vi "000Main V180214.vi"() -> ()   [LabVIEW 2015]
uses:
  0254/BrooksDLL64.dll
panel:
  out "Function Output Comment 4":string
  out "output param 4":i32
  out "Function Output Comment 3":string
  out "output param 3":i32
  in  "0254 Decimal Place 3":i32(ring) items=["xxx.", "xx.x", "x.xx", ".xxx"]
  out "Function Output Comment 5":string
  out "output param 5":i32
  in  "0254 Decimal Place 4":i32(ring) items=["xxx.", "xx.x", "x.xx", ".xxx"]
  out "Function Output Comment 6":string
  out "output param 6":i32
  out "resistance":cluster{dbl[], dbl[]}(graph)
  out "current":cluster{dbl[], dbl[]}(graph)
  out "flow2":cluster{dbl[], dbl[]}(graph)
  in  "?":enum32{"initialization", "step", "other"}(tab)
  in  "Start_2400":bool
  in  "Delay (ms)":u32=1000
  in  "Target (V)":dbl=0.1
  in  "Step (V)":dbl=0.005
  in  "Stop":bool
  in  "file path (use dialog)":path
  in  "?":bool
  in  "sum flow 2":dbl=100.0 format="%#_13g"
  in  "VISA 0254":refnum<visa-resource-name>
  in  "VISA 2400":refnum<visa-resource-name>
  in  "Gas Flow Enable":bool
  in  "flow2 1":dbl=100.0 format="%#_13g"
  in  "time1":dbl=1000.0 format="%#_13g"
  in  "flow2 2":dbl format="%#_13g"
  in  "time2":dbl=1000.0 format="%#_13g"
  in  "flow2 3":dbl=100.0 format="%#_13g"
  in  "time3":dbl=1000.0 format="%#_13g"
  in  "time4":dbl=1000.0 format="%#_13g"
  out "voltage":string
  out "Current":dbl
  out "Time (s)":dbl
  out "flow1":sgl format="%.2f"
  out "flow2":sgl format="%.2f"
  out "Initiliazation Started":bool
  in  "Initialization":bool
  # "flow2 = 0"
  # "flow2 = 0"
  # "time   voltage  current  flow1  flow2  resistance"
  # "Please Wait  ~ 25 s"
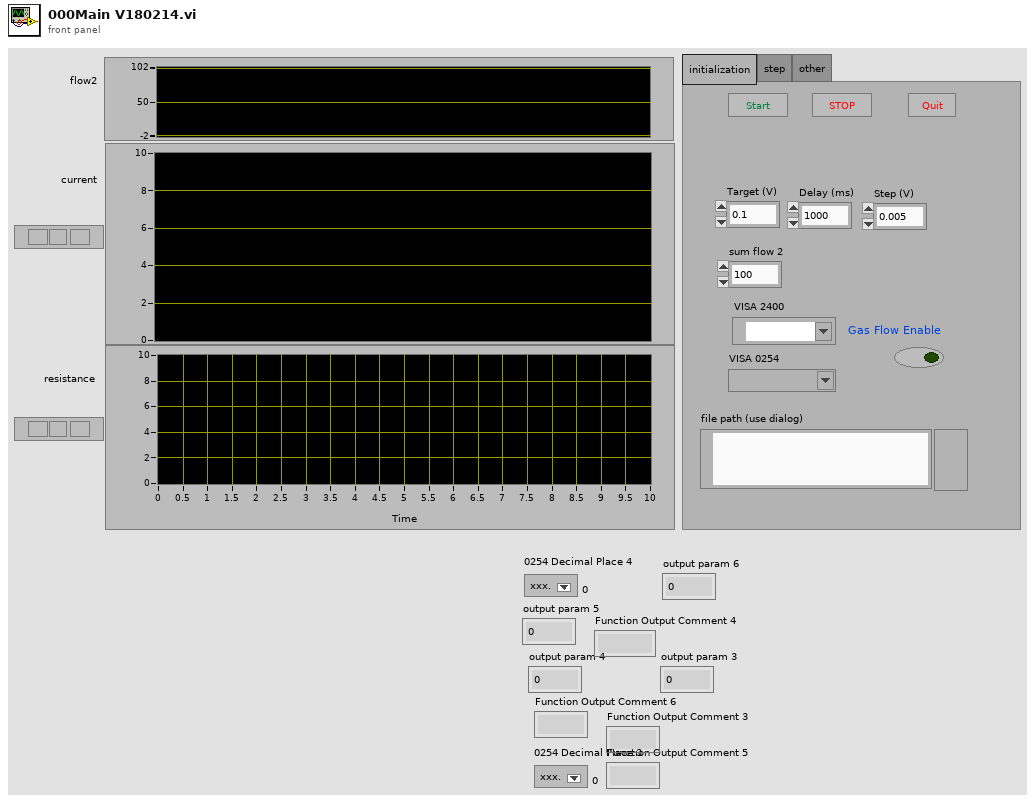
[diagram p1: front panel]
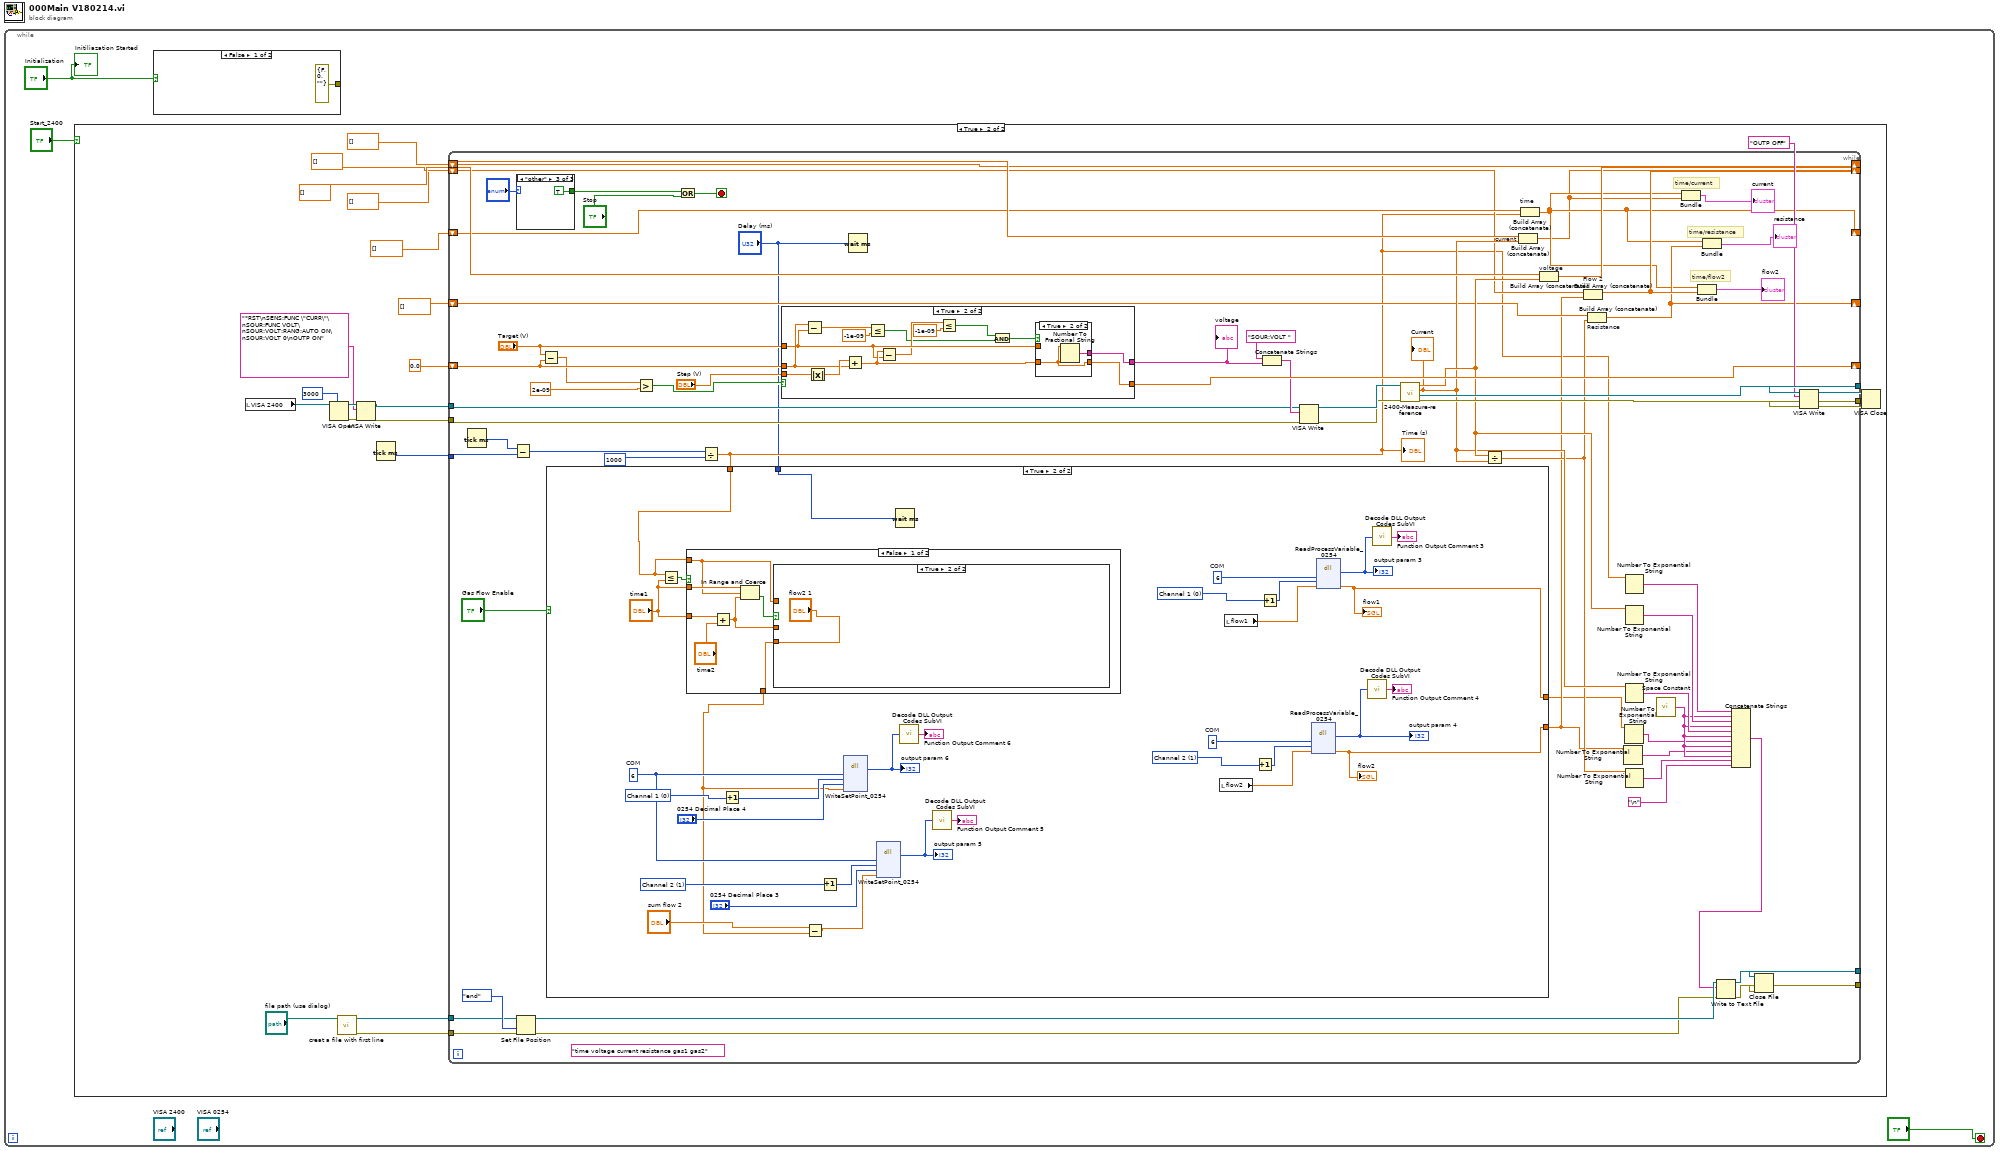
[diagram p0: block diagram]
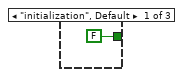
[diagram p3: hidden frame]
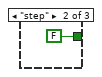
[diagram p4: hidden frame]
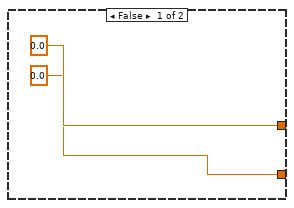
[diagram p5: hidden frame]
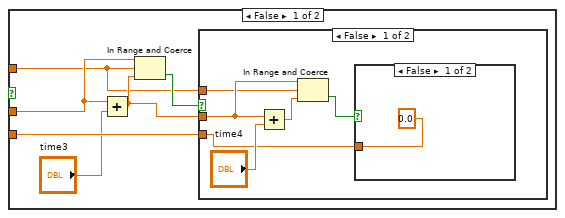
[diagram p6: hidden frame]
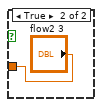
[diagram p7: hidden frame]
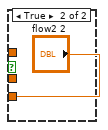
[diagram p8: hidden frame]
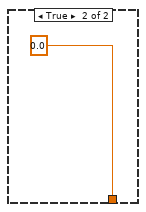
[diagram p9: hidden frame]
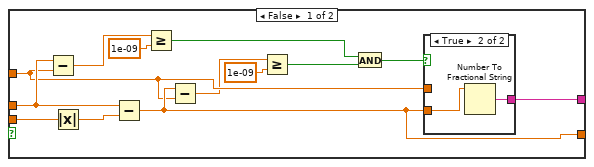
[diagram p10: hidden frame]
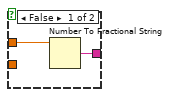
[diagram p11: hidden frame]
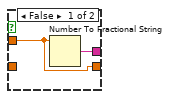
[diagram p12: hidden frame]
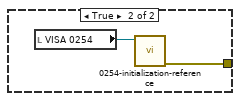
[diagram p13: hidden frame]
diagram:
  n1 = while {
    stop <- "?" stop-if-true
    n2 = case shown="True" "Start_2400" {
      frame False {
      }
      frame True {
        n3 = local read "VISA 2400"() -> (w20:refnum<visa-resource-name>)
        n4 = VISA Open(timeout (0)=3000 ("timeout ms (488.2 global)"), VISA resource name=w20) -> (VISA resource name=w23:refnum<visa-resource-name>, error out=w22:errorcluster)  [unwired: 3 in]
        n5 = call "creat a file with first line.vi"("file path (use dialog)"="file path (use dialog)") -> ("error out"=w5:errorcluster, "Byte Stream File out"=w6:refnum<file>)  [unwired: 9 in]
        n6 = VISA Write(VISA resource name=w23, write buffer="*RST\nSENS:FUNC \"CURR\"\nSOUR:FUNC VOLT\nSOUR:VOLT:RANG:AUTO ON\nSOUR:VOLT 0\nOUTP ON" ("data"), error in (no error)=w22) -> (VISA resource name out=w17:refnum<visa-resource-name>, error out=w18:errorcluster)  [unwired: 1 out]
        n7 = Tick Count (ms)() -> (millisecond timer value=w4:u32)
        n8 = while {
          shift-right: [w80] -> _
          shift-left: 0.0 ("Target (V)") -> [w76]
          shift-right: [w47] -> _
          shift-left: dbl[] [] -> [w89]
          shift-right: [w42] -> _
          shift-left: dbl[] [] -> [w88]
          tunnel: w6 -> [w41]
          tunnel: w5 -> [w85]
          tunnel: [w65] -> w26
          tunnel: [w50] -> w25
          tunnel: w17 -> [w72]
          tunnel: [w61] -> w13
          tunnel: [w60] -> w12
          tunnel: w18 -> [w66]
          tunnel: w4 -> [w37]
          shift-right: [w43] -> _
          shift-left: dbl[] [] -> [w67]
          shift-right: [w48] -> _
          shift-left: dbl[] [] -> [w49]
          shift-right: [w46] -> _
          shift-left: dbl[] [] -> [w46]
          shift-right: [w44] -> _
          shift-left: dbl[] [] -> [w45]
          stop <- w55 stop-if-true
          (unwired) "time voltage current resistance gas1 gas2"
          # "time/flow2"
          # "time/resistance"
          # "time/current"
          n9 = Tick Count (ms)() -> (millisecond timer value=w70:u32)
          n10 = Subtract(x=w70, y=w37) -> (x-y=w69:u32)
          n11 = case shown="\"other\"" "?" {
            tunnel: [FALSE FALSE TRUE] -> w57
            frame "initialization", Default {
            }
            frame "step" {
            }
            frame "other" {
            }
          }
          n12 = Set File Position(refnum=w41, from (0:start)=enum16{"start", "end", "current"}."end", error in=w85) -> (refnum out=w84:refnum<file>, error out=w83:errorcluster)  [unwired: 1 out]
          n13 = Subtract(x="Target (V)", y=w76) -> (x-y=w75:dbl)
          n14 = Greater?(x=w75, y=2e-09) -> (0:w79:bool)
          n15 = Or(x=w57, y="Stop") -> (x .or. y?=w55:bool)
          n16 = Divide(x=w69, y=u32 1000) -> (x/y=w33:dbl)
          "Time (s)" <- w33
          n17 = case shown="True" "Gas Flow Enable" {
            tunnel: [sgl 0.0 ("PV") w126] -> w35
            tunnel: [sgl 0.0 ("PV") w127] -> w34
            tunnel: w33 -> [_ w125]
            tunnel: "Delay (ms)" -> [_ w96]
            frame False {
            }
            frame True {
              w99 = 1 items=["Channel 1", "Channel 2", "Channel 3", "Channel 4"] ("0254 Channel (1-4)")
              w103 = 6  # COM
              w105 = 0 items=["Channel 1", "Channel 2", "Channel 3", "Channel 4"] ("0254 Channel (1-4)")
              w109 = 6  # COM
              w122 = 0 items=["Channel 1", "Channel 2", "Channel 3", "Channel 4"] ("0254 Channel (1-4)")
              w118 = 1 items=["Channel 1", "Channel 2", "Channel 3", "Channel 4"] ("0254 Channel 2")
              w113 = 6  # COM
              n18 = Less Or Equal?(x=w125, y="time1") -> (x <= y?=w110:bool)
              n19 = case shown="False" w110 {
                tunnel: [w132 0.0 ("flow2 2")] -> w111
                tunnel: w125 -> [w130 _]
                tunnel: "time1" -> [w134 _]
                tunnel: "time1" -> [w128 _]
                frame False {
                  n20 = Add(x=w128, y="time2") -> (x+y=w129:dbl)
                  n21 = In Range and Coerce(upper limit=w134, x=w130, lower limit=w129) -> (In Range?=w133:bool)  [unwired: 1 out]
                  n22 = case shown="True" w133 {
                    tunnel: [w139 "flow2 1"] -> w132
                    tunnel: w130 -> [w135 _]
                    tunnel: w129 -> [w138 _]
                    frame False {
                      n23 = Add(x=w138, y="time3") -> (x+y=w136:dbl)
                      n24 = In Range and Coerce(upper limit=w138, x=w135, lower limit=w136) -> (In Range?=w140:bool)  [unwired: 1 out]
                      n25 = case shown="False" w140 {
                        tunnel: [w141 "flow2 2"] -> w139
                        tunnel: w136 -> [w144 _]
                        tunnel: w135 -> [w143 _]
                        frame False {
                          n26 = Add(x=w144, y="time4") -> (x+y=w145:dbl)
                          n27 = In Range and Coerce(upper limit=w144, x=w143, lower limit=w145) -> (In Range?=w142:bool)  [unwired: 1 out]
                          n28 = case shown="False" w142 {
                            tunnel: [0.0 "flow2 3"] -> w141
                            frame False {
                            }
                            frame True {
                            }
                          }
                        }
                        frame True {
                        }
                      }
                    }
                    frame True {
                    }
                  }
                }
                frame True {
                }
              }
              n29 = Increment(x=w122) -> (x+1=w123:i32)
              n30 = Subtract(x="sum flow 2", y=w111) -> (x-y=w115:dbl)
              n31 = Increment(x=w118) -> (x+1=w119:i32)
              n32 = dll-call lib="C:/Users/Atom/Desktop/gas test V180214 for LV12/0254/BrooksDLL64.dll" fn="WriteSetPoint_0254"("COM"=w113, "Channel"=w123, "DP"="0254 Decimal Place 4", "SetPoint"=w111) -> ("return type"=w112:i32)  [unwired: 7 in, 2 out]
              "output param 6" <- w112
              n33 = dll-call lib="C:/Users/Atom/Desktop/gas test V180214 for LV12/0254/BrooksDLL64.dll" fn="WriteSetPoint_0254"("COM"=w113, "Channel"=w119, "DP"="0254 Decimal Place 3", "SetPoint"=w115) -> ("return type"=w116:i32)  [unwired: 7 in, 2 out]
              "output param 5" <- w116
              n34 = Wait (ms)(milliseconds to wait=w96) -> ()  [unwired: 1 out]
              n35 = call "Decode DLL Output Codes SubVI.vi"("Numeric"=w112) -> ("Function Output Comment"=→"Function Output Comment 6":string)
              n36 = call "Decode DLL Output Codes SubVI.vi"("Numeric"=w116) -> ("Function Output Comment"=→"Function Output Comment 5":string)
              n37 = local read "flow2"() -> (w100:sgl)
              n38 = local read "flow1"() -> (w106:sgl)
              n39 = Increment(x=w99) -> (x+1=w98:i32)
              n40 = Increment(x=w105) -> (x+1=w104:i32)
              n41 = dll-call lib="C:/Users/Atom/Desktop/gas test V180214 for LV12/0254/BrooksDLL64.dll" fn="ReadProcessVariable_0254"("COM"=w103, "Channel"=w98, "PV"=w100) -> ("return type"=w102:i32, "PV"=w126:sgl)  [unwired: 5 in, 2 out]
              "output param 4" <- w102
              "flow2" <- w126
              n42 = dll-call lib="C:/Users/Atom/Desktop/gas test V180214 for LV12/0254/BrooksDLL64.dll" fn="ReadProcessVariable_0254"("COM"=w109, "Channel"=w104, "PV"=w106) -> ("return type"=w108:i32, "PV"=w127:sgl)  [unwired: 5 in, 2 out]
              "output param 3" <- w108
              "flow1" <- w127
              n43 = call "Decode DLL Output Codes SubVI.vi"("Numeric"=w102) -> ("Function Output Comment"=→"Function Output Comment 4":string)
              n44 = call "Decode DLL Output Codes SubVI.vi"("Numeric"=w108) -> ("Function Output Comment"=→"Function Output Comment 3":string)
            }
          }
          n45 = case shown="True" w79 {
            tunnel: "Step (V)" -> [w164 w182]
            tunnel: w76 -> [w159 w177]
            tunnel: "Target (V)" -> [w158 w176]
            tunnel: [w161 w179] -> w80
            tunnel: [w160 w178] -> w78
            frame False {
              n46 = Subtract(x=w159, y=w158) -> (x-y=w152:dbl)
              n47 = Absolute Value(x=w164) -> (abs(x)=w163:dbl)
              n48 = Subtract(x=w159, y=w163) -> (x-y=w161:dbl)
              n49 = Greater Or Equal?(x=w152, y=1e-09) -> (x >= y?=w156:bool)
              n50 = Subtract(x=w161, y=w158) -> (x-y=w153:dbl)
              n51 = Greater Or Equal?(x=w153, y=1e-09) -> (x >= y?=w155:bool)
              n52 = And(x=w156, y=w155) -> (x .and. y?=w154:bool)
              n53 = case shown="True" w154 {
                tunnel: w161 -> [_ w168]
                tunnel: [w165 w167] -> w160
                tunnel: w158 -> [w166 _]
                frame False {
                  n54 = Number To Fractional String(number=w166) -> (F-format string=w165:string)  [unwired: 3 in]
                }
                frame True {
                  n55 = Number To Fractional String(number=w168) -> (F-format string=w167:string)  [unwired: 3 in]
                }
              }
            }
            frame True {
              n56 = Subtract(x=w177, y=w176) -> (x-y=w171:dbl)
              n57 = Absolute Value(x=w182) -> (abs(x)=w181:dbl)
              n58 = Add(x=w181, y=w177) -> (x+y=w180:dbl)
              n59 = Less Or Equal?(x=w171, y=-1e-09) -> (x <= y?=w169:bool)
              n60 = Subtract(x=w180, y=w176) -> (x-y=w174:dbl)
              n61 = Less Or Equal?(x=w174, y=-1e-09) -> (x <= y?=w172:bool)
              n62 = And(x=w172, y=w169) -> (x .and. y?=w175:bool)
              n63 = case shown="True" w175 {
                tunnel: w180 -> [_ w185]
                tunnel: [w184 w186] -> w178
                tunnel: w176 -> [w183 _]
                tunnel: [w183 w185] -> w179
                frame False {
                  n64 = Number To Fractional String(number=w183) -> (F-format string=w184:string)  [unwired: 3 in]
                }
                frame True {
                  n65 = Number To Fractional String(number=w185) -> (F-format string=w186:string)  [unwired: 3 in]
                }
              }
            }
          }
          "voltage" <- w78
          n66 = Wait (ms)(milliseconds to wait="Delay (ms)") -> ()  [unwired: 1 out]
          n67 = Concatenate Strings("SOUR:VOLT " ("string"), w78) -> (w73:string)
          n68 = VISA Write(VISA resource name=w72, write buffer=w73, error in (no error)=w66) -> (VISA resource name out=w63:refnum<visa-resource-name>, error out=w62:errorcluster)  [unwired: 1 out]
          n69 = call "2400-Measure-reference.vi"("error in (no error)"=w62, "VISA Refnum in"=w63) -> ("error out"=w60:errorcluster, "VISA resource name out"=w61:refnum<visa-resource-name>, "Current Output"=w51:dbl, "Voltage Output"=w52:dbl)  [unwired: 6 in]
          "Current" <- w51
          n70 = Divide(x=w52, y=w51) -> (x/y=w36:dbl)
          n71 = Build Array (concatenate) "current"(w88, w51) -> (w42:dbl[])
          n72 = Build Array (concatenate) "time"(w67, w33) -> (w43:dbl[])
          n73 = Build Array (concatenate) "voltage"(w89, w52) -> (w47:dbl[])
          n74 = Build Array (concatenate) "Flow 2"(w49, w35) -> (w48:dbl[])
          n75 = Build Array (concatenate) "Resistance"(w45, w36) -> (w44:dbl[])
          n76 = Number To Exponential String(number=w35) -> (E-format string=w38:string)  [unwired: 3 in]
          n77 = Number To Exponential String(number=w34) -> (E-format string=w40:string)  [unwired: 3 in]
          n78 = Number To Exponential String(number=w33) -> (E-format string=w68:string)  [unwired: 3 in]
          n79 = Number To Exponential String(number=w52) -> (E-format string=w86:string)  [unwired: 3 in]
          n80 = Number To Exponential String(number=w51) -> (E-format string=w87:string)  [unwired: 3 in]
          n81 = Number To Exponential String(number=w36) -> (E-format string=w39:string)  [unwired: 3 in]
          n82 = call <vilib>:"Space Constant.vi"() -> ("String"=w54:string)
          n83 = Bundle(w43, w42) -> (→"current":cluster{dbl[], dbl[]})  [unwired: 1 in]
          n84 = Bundle(w43, w48) -> (→"flow2":cluster{dbl[], dbl[]})  [unwired: 1 in]
          n85 = Bundle(w43, w44) -> (→"resistance":cluster{dbl[], dbl[]})  [unwired: 1 in]
          n86 = Concatenate Strings(w68, w54, w86, w54, w87, w54, w40, w54, w38, w54, w39, "\n") -> (w64:string)
          n87 = Write to Text File(file (use dialog)=w84, text=w64, error in=w83) -> (refnum out=w50:refnum<file>, error out=w65:errorcluster)  [unwired: 1 in, 1 out]
        }
        n88 = Close File(refnum=w25, error in=w26) -> ()  [unwired: 2 out]
        n89 = VISA Write(VISA resource name=w13, write buffer="OUTP OFF" ("data"), error in (no error)=w12) -> (VISA resource name out=w15:refnum<visa-resource-name>, error out=w14:errorcluster)  [unwired: 1 out]
        n90 = VISA Close(VISA resource name=w15, error in (no error)=w14) -> ()  [unwired: 1 out]
      }
    }
    n91 = case shown="False" "Initialization" {
      tunnel: [errorcluster {"status"=FALSE, "code"=0, "source"=""} ("error out") w188] -> _
      frame False {
      }
      frame True {
        n92 = local read "VISA 0254"() -> (w189:refnum<visa-resource-name>)
        n93 = call "0254-initialization-reference.vi"("0254-VISA"=w189) -> ("error out"=w188:errorcluster)  [unwired: 8 in, 2 out]
      }
    }
    "Initiliazation Started" <- "Initialization"
  }
